vi "Process Channel.vi"(0 "Software Lock-in in":refnum<class "Software Lock-in.lvclass">, 1 "tdms file":refnum<k34>, 2 "Phase":dbl, 5 "Group name":string, 9 "Channel name":string, 11 "error in (no error)":errorcluster, 12 "Time constant":dbl, 13 "Harmonic":i32=1) -> (3 "tdms file out":refnum<k34>, 4 "Software Lock-in out":refnum<class "Software Lock-in.lvclass">, 6 "Signal":dynamicdata(graph), 8 "Time axis":dbl[](array[numeric]), 10 "Channel names":string[](array[string]), 14 "dt":dbl, 15 "error out":errorcluster)   [LabVIEW 2016, in "Software Lock-in.lvclass"]
uses:
  Software Lock-in.lvclass
  Software Lock-in.lvclass/Software Lock-in.ctl
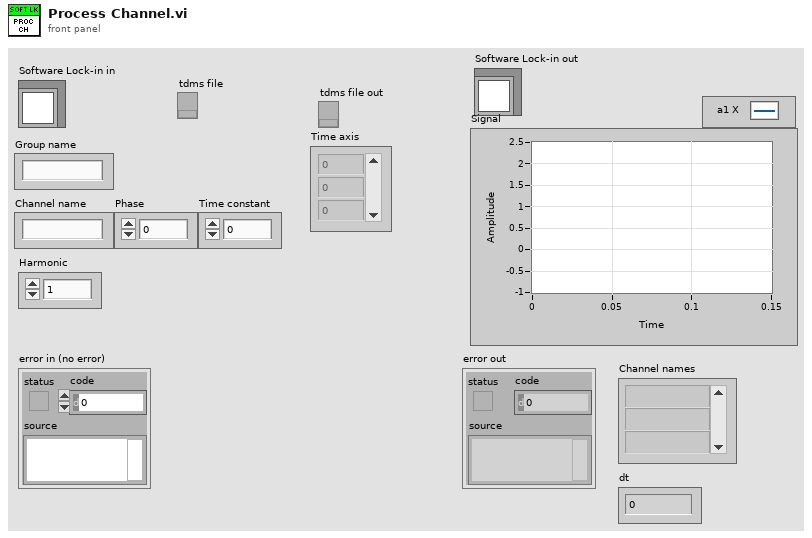
[diagram p1: front panel]
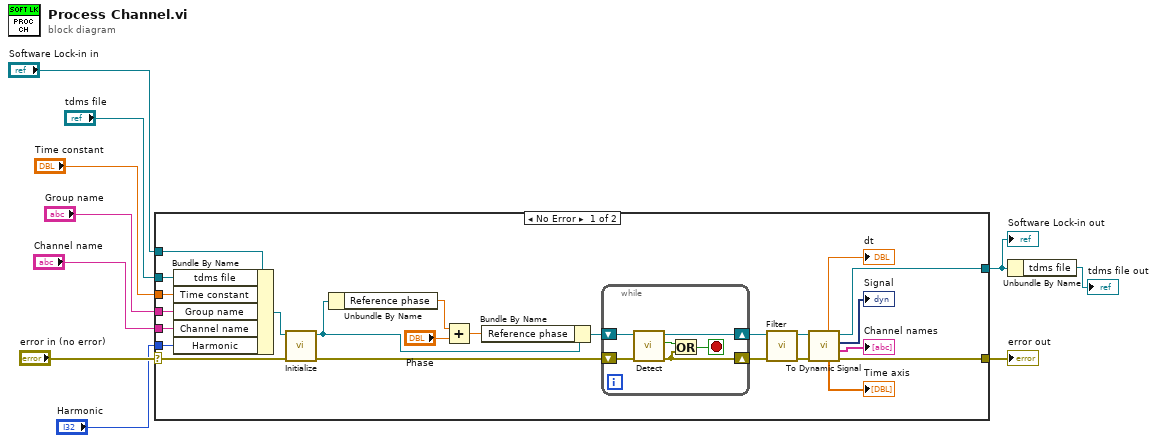
[diagram p0: block diagram]
diagram:
  n1 = case shown="No Error" "error in (no error)" {
    selector: "error in (no error)" -> [w33 w42]
    tunnel: [w20 w42] -> w9
    tunnel: [w22 w41] -> w7
    tunnel: "Software Lock-in in" -> [w34 w41]
    tunnel: "Harmonic" -> [w15 _]
    tunnel: "Channel name" -> [w14 _]
    tunnel: "Group name" -> [w13 _]
    tunnel: "Time constant" -> [w12 _]
    tunnel: "tdms file" -> [w11 _]
    frame No Error {
      n2 = Bundle By Name(cluster=w34, "tdms file"=w11, "Time constant"=w12, "Group name"=w13, "Channel name"=w14, "Harmonic"=w15) -> (w24:refnum<class "Software Lock-in.lvclass">)
      n3 = call-dynamic "Initialize.vi"("error in (no error)"=w33, "Software Lock-in in"=w24) -> ("error out"=w32:errorcluster, "Software Lock-in out"=w31:refnum<class "Software Lock-in.lvclass">)  [unwired: 8 in]
      n4 = Unbundle By Name(w31) -> ("Reference phase"=w30:dbl)
      n5 = Add(x=w30, y="Phase") -> (x+y=w27:dbl)
      n6 = Bundle By Name(cluster=w31, "Reference phase"=w27) -> (w28:refnum<class "Software Lock-in.lvclass">)
      n7 = while {
        shift-right: [w38] -> w26
        shift-left: w28 -> [w40]
        shift-right: [w35] -> w25
        shift-left: w32 -> [w37]
        stop <- w36 stop-if-true
        n8 = call-dynamic "Detect.vi"("error in (no error)"=w37, "Software Lock-in in"=w40) -> ("error out"=w35:errorcluster, "Finished"=w39:bool, "Software Lock-in out"=w38:refnum<class "Software Lock-in.lvclass">)  [unwired: 7 in]
        n9 = Or(x=w39, y=w35) -> (x .or. y?=w36:bool)
      }
      n10 = call-dynamic "Filter.vi"("error in (no error)"=w25, "Software Lock-in in"=w26) -> ("error out"=w21:errorcluster, "Software Lock-in out"=w23:refnum<class "Software Lock-in.lvclass">)  [unwired: 8 in]
      n11 = call "To Dynamic Signal.vi"("error in (no error)"=w21, "Software Lock-in in"=w23) -> ("error out"=w20:errorcluster, "Channel names"=→"Channel names":string[], "Signal"=→"Signal":dynamicdata, "Software Lock-in out"=w22:refnum<class "Software Lock-in.lvclass">, "Time axis"=→"Time axis":dbl[], "dt"=→"dt":dbl)  [unwired: 4 in]
    }
    frame Error {
    }
  }
  "error out" <- w9
  "Software Lock-in out" <- w7
  n12 = Unbundle By Name(w7) -> ("tdms file"=→"tdms file out":refnum<k34>)
